vi "Radiometer_calibration.vi"(2 "V_2":dbl=1.561099753965909 caption="High\nVoltage (mV)" step=0.001 format="%#_3g", 3 "T_2":dbl=60.0 caption="High\nTemperature (C)", 4 "V_1":dbl=0.08625226405498748 caption="Low\nVoltage (mV)" step=0.001 format="%#_3g", 5 "T_1":dbl=21.0 caption="Low\nTemperature (C)") -> (0 "b=T_2+a*V_2":dbl caption="Const - b" format="%#_5g", 1 "a=(T_2-T_1)/(V_2-V_1)":dbl caption="Slope - a" format="%#_5g")   [LabVIEW 2017]
doc: "This VI will find the coefficients of the linear transformation V=a*T+b.\nIt will use two (T,V) pairs to calculate a and b.\nAll inputs are optional and they are the values of Thigh, Tlow, Vhigh and Vlow. These values can be determaind while the VI is running.\nThis VI is teminated when \"CALIBRATE\" button is pressed. The VI's output is the a and b coefficients."
uses:
  DAQmx Create Channel (AI-Voltage-Basic).vi
  <vilib>/Utility/error.llb/DialogType.ctl
  DAQmx Read (Analog 1D DBL NChan 1Samp).vi
panel:
  in  "Rad. channel 2":tag="Dev1/ai3" caption="rad channel ai0"
  in  "RadB factor":dbl
  out "Temp":dbl=18.637306869936005 caption="Calibrated\nTeperature" format="%#_3g"
  in  "btn_COPY_HIGH":bool
  in  "btn_COPY_LOW":bool
  out "cur reading":dbl=-0.00309676241436279 caption="Current\nReading" format="%#_3g"
  in  "stop":bool
  out "Formula":string="T= 26.443 *V+ 18.719" caption="Radiometer Calibration"
  # "Radiometer Calibration"
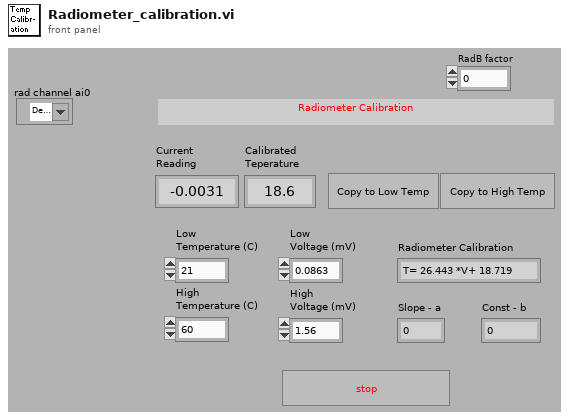
[diagram p1: front panel]
types:
  T1 = typedef "DialogType.ctl" = u16
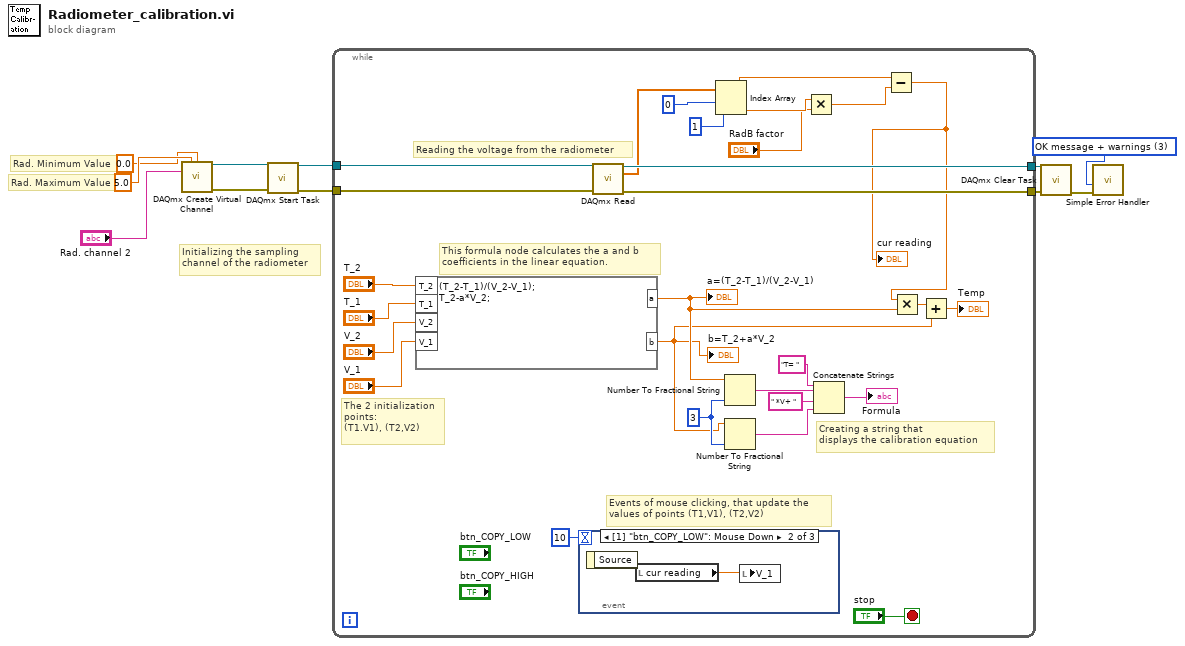
[diagram p0: block diagram]
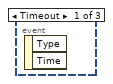
[diagram p2: hidden frame]
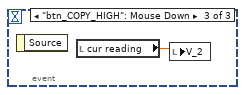
[diagram p3: hidden frame]
diagram:
  w11 = T1 3 items=["no dialog", "OK message", "continue or stop message", "OK message + warnings", "continue/stop + warnings"] ("type of dialog (OK msg:1)")
  # "Initializing the sampling \nchannel of the radiometer"
  # "Rad. Maximum Value"
  # "Rad. Minimum Value"
  n1 = call-poly "DAQmx Create Virtual Channel.vi"("maximum value"=5.0 ("Rad. Maximum Value"), "minimum value"=0.0 ("Rad. Minimum Value"), "physical channels"="Rad. channel 2") -> ("task out"=w8:refnum<k21>, "error out"=w9:errorcluster)  [unwired: 11 in]
  n2 = call "DAQmx Start Task.vi"("task/channels in"=w8, "error in"=w9) -> ("task out"=w5:refnum<k21>, "error out"=w4:errorcluster)  [unwired: 12 in]
  n3 = while {
    tunnel: w5 -> [w24]
    tunnel: w4 -> [w23]
    tunnel: [w22] -> w3
    tunnel: [w21] -> w2
    stop <- "stop" stop-if-true
    w34 = i16 3 ("precision (6)")
    # "Creating a string that \ndisplays the calibration equation"
    # "Reading the voltage from the radiometer"
    # "The 2 initialization \npoints: \n(T1.V1), (T2,V2)"
    # "Events of mouse clicking, that update the \nvalues of points (T1,V1), (T2,V2)"
    # "This formula node calculates the a and b \ncoefficients in the linear equation."
    n4 = formula code="a=(T_2-T_1)/(V_2-V_1);\nb=T_2-a*V_2;"("T_2"="T_2", "T_1"="T_1", "V_2"="V_2", "V_1"="V_1") -> ("a"=w27:dbl, "b"=w20:dbl)
    "a=(T_2-T_1)/(V_2-V_1)" <- w27
    "b=T_2+a*V_2" <- w20
    n5 = event shown="[1] \"btn_COPY_LOW\": Mouse Down" {
      selector: _ -> [_ _ _]
      dyn-events: _ -> [_ _ _]
      timeout: 10 -> [_ _ _]
      event Timeout {
        n6 = event-data() -> ()  [unwired: 1 in, 2 out]
      }
      event "btn_COPY_LOW": Mouse Down {
        n7 = event-data() -> ()  [unwired: 1 in, 1 out]
        n8 = local read "cur reading"() -> (w40:dbl)
        n9 = local write "V_1"(w40) -> ()
      }
      event "btn_COPY_HIGH": Mouse Down {
        n10 = event-data() -> ()  [unwired: 1 in, 1 out]
        n11 = local read "cur reading"() -> (w41:dbl)
        n12 = local write "V_2"(w41) -> ()
      }
    }
    n13 = call-poly "DAQmx Read.vi"("task/channels in"=w24, "error in"=w23) -> ("task out"=w22:refnum<k21>, "data"=w17:dbl[], "error out"=w21:errorcluster)  [unwired: 11 in]
    n14 = Index Array(array=w17, index #1=0 ("index"), index #2=1 ("index")) -> (element #1=w16:dbl, element #2=w13:dbl)
    n15 = Number To Fractional String(number=w27, precision (6)=w34) -> (F-format string=w38:string)  [unwired: 2 in]
    n16 = Number To Fractional String(number=w20, precision (6)=w34) -> (F-format string=w36:string)  [unwired: 2 in]
    n17 = Multiply(x=w13, y="RadB factor") -> (x*y=w14:dbl)
    n18 = Concatenate Strings("T= " ("string"), w38, " *V+ " ("string"), w36) -> (→"Formula":string)
    n19 = Subtract(x=w16, y=w14) -> (x-y=w15:dbl)
    "cur reading" <- w15
    n20 = Multiply(x=w15, y=w27) -> (x*y=w26:dbl)
    n21 = Add(x=w26, y=w20) -> (x+y=→"Temp":dbl)
  }
  n22 = call "DAQmx Clear Task.vi"("task in"=w3, "error in"=w2) -> ("error out"=w10:errorcluster)  [unwired: 13 in]
  n23 = call <vilib>:"Simple Error Handler.vi"("type of dialog (OK msg:1)"=w11, "error in (no error)"=w10) -> ()  [unwired: 3 in, 5 out]
